vi "Write Last  Statusword.vi"(8 "error in (no error)":errorcluster, 10 "Statusword":T1, 11 "Motor Base in":refnum<class "Motor Base.lvclass">) -> (0 "error out":errorcluster, 3 "Motor Base out":refnum<class "Motor Base.lvclass">)   [LabVIEW 2016, in "Motor Base.lvlib" / "Motor Base.lvclass"]
uses:
  Motor Base.lvclass
  PDS/Statusword.ctl
  Motor Base.lvclass/Motor Base.ctl
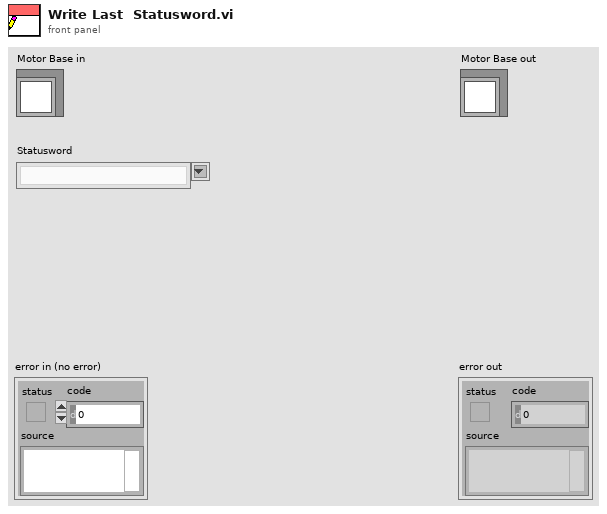
[diagram p1: front panel]
types:
  T1 = typedef "Motor Base.lvlib/Motor Base.lvclass/Statusword.ctl" = string
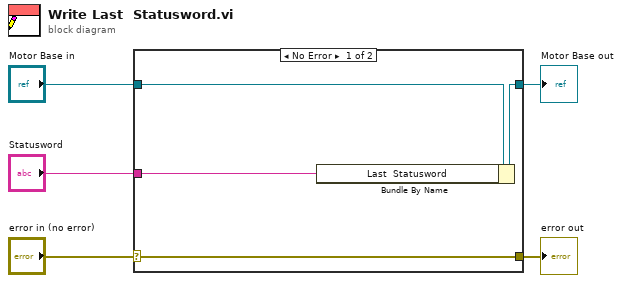
[diagram p0: block diagram]
diagram:
  n1 = case shown="No Error" "error in (no error)" {
    selector: "error in (no error)" -> [w9 w10]
    tunnel: [w9 w10] -> w4
    tunnel: [w7 w11] -> w2
    tunnel: "Motor Base in" -> [w8 w11]
    tunnel: "Statusword" -> [w6 _]
    frame No Error {
      n2 = Bundle By Name(cluster=w8, "Last  Statusword"=w6) -> (w7:refnum<class "Motor Base.lvclass">)
    }
    frame Error {
    }
  }
  "error out" <- w4
  "Motor Base out" <- w2
